vi "parse core.vi"(11 "URL":string) -> (0 "query":string, 1 "path":string, 2 "port":string, 3 "host":string, 4 "password":string, 5 "username":string, 6 "fragment":string, 7 "scheme":string)   [LabVIEW 2013, in "uniform resource locator.lvlib"]
uses:
  uniform resource locator.lvlib
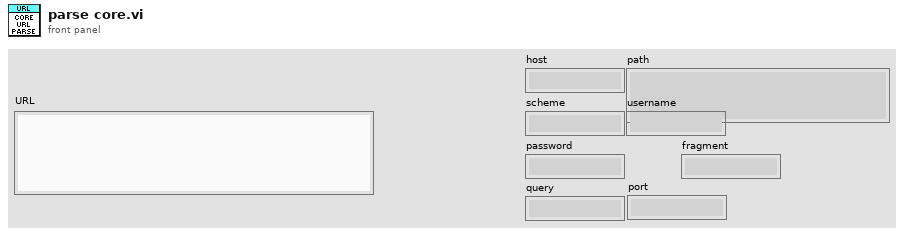
[diagram p1: front panel]
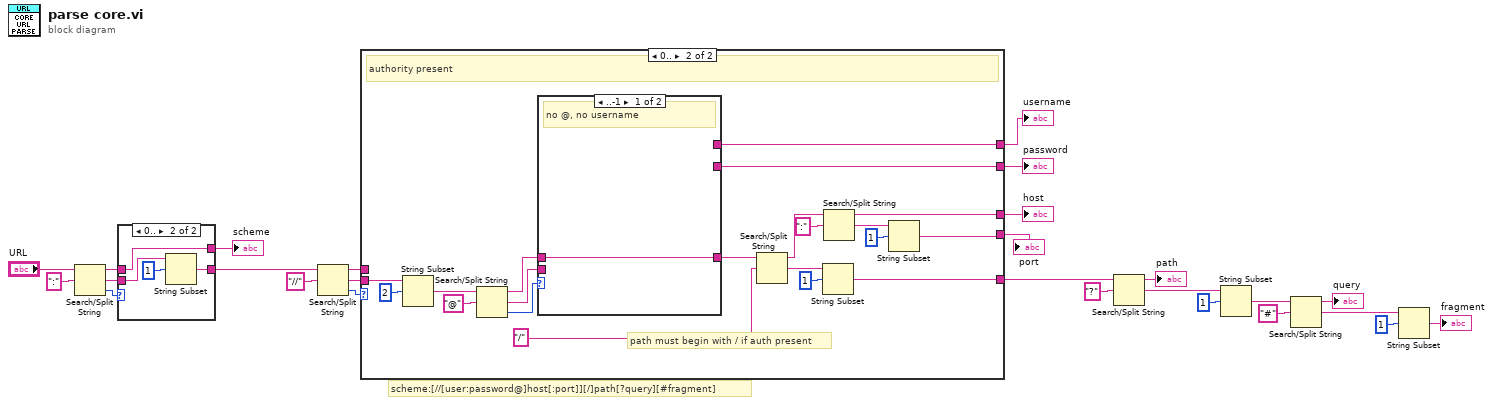
[diagram p0: block diagram]
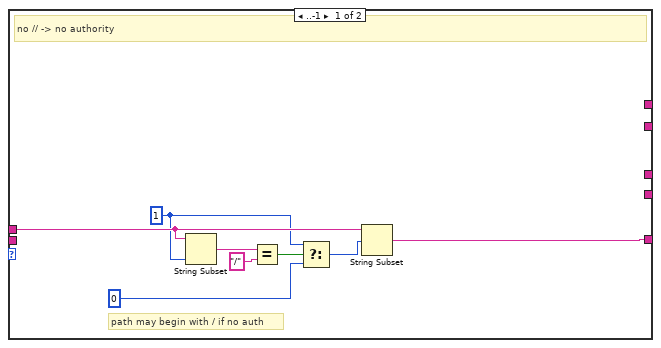
[diagram p2: hidden frame]
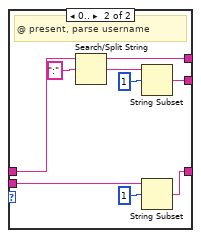
[diagram p3: hidden frame]
diagram:
  # "scheme:[//[user:password@]host[:port]][/]path[?query][#fragment]"
  n1 = Search/Split String(string="URL", search string/char (-)=":" ("regular expression")) -> (substring before match=w22:string, match + rest of string=w21:string, offset of match=w24:i32)  [unwired: 1 in]
  n2 = case shown="0.." w24 {
    tunnel: [_ w31] -> w23
    tunnel: w22 -> [w27 w31]
    tunnel: [w27 w29] -> w17
    tunnel: w21 -> [_ w30]
    frame ..-1 {
    }
    frame 0.. {
      n3 = String Subset(string=w30, offset (0)=1) -> (substring=w29:string)  [unwired: 1 in]
    }
  }
  "scheme" <- w23
  n4 = Search/Split String(string=w17, search string/char (-)="//" ("regular expression")) -> (substring before match=w19:string, match + rest of string=w20:string, offset of match=w16:i32)  [unwired: 1 in]
  n5 = case shown="0.." w16 {
    tunnel: w20 -> [_ w59]
    tunnel: w19 -> [w37 _]
    tunnel: [_ w44] -> w15
    tunnel: [w36 w47] -> w9
    tunnel: [_ w52] -> w14
    tunnel: [_ w51] -> w13
    tunnel: [_ w40] -> w1
    frame ..-1 {
      w34 = 1 ("length (rest)")
      # "path may begin with / if no auth"
      # "no // -> no authority"
      n6 = String Subset(string=w37, length (rest)=w34) -> (substring=w39:string)  [unwired: 1 in]
      n7 = Equal?(x=w39, y="/" ("regular expression")) -> (x = y?=w35:bool)
      n8 = Select(t=w34, s=w35, f=0) -> (s? t:f=w32:i32)
      n9 = String Subset(string=w37, offset (0)=w32) -> (substring=w36:string)  [unwired: 1 in]
    }
    frame 0.. {
      # "path must begin with / if auth present"
      # "authority present"
      n10 = String Subset(string=w59, offset (0)=2) -> (substring=w54:string)  [unwired: 1 in]
      n11 = Search/Split String(string=w54, search string/char (-)="@" ("regular expression")) -> (substring before match=w56:string, match + rest of string=w55:string, offset of match=w57:i32)  [unwired: 1 in]
      n12 = case shown="..-1" w57 {
        tunnel: w56 -> [w60 w64]
        tunnel: [w60 w68] -> w48
        tunnel: w55 -> [_ w69]
        tunnel: [_ w62] -> w52
        tunnel: [_ w61] -> w51
        frame ..-1 {
          # "no @, no username"
        }
        frame 0.. {
          # "@ present, parse username"
          n13 = Search/Split String(string=w64, search string/char (-)=":" ("regular expression")) -> (substring before match=w62:string, match + rest of string=w66:string)  [unwired: 1 in, 1 out]
          n14 = String Subset(string=w66, offset (0)=1) -> (substring=w61:string)  [unwired: 1 in]
          n15 = String Subset(string=w69, offset (0)=1) -> (substring=w68:string)  [unwired: 1 in]
        }
      }
      n16 = Search/Split String(string=w48, search string/char (-)="/" ("regular expression")) -> (substring before match=w42:string, match + rest of string=w50:string)  [unwired: 1 in, 1 out]
      n17 = String Subset(string=w50, offset (0)=1) -> (substring=w47:string)  [unwired: 1 in]
      n18 = Search/Split String(string=w42, search string/char (-)=":" ("regular expression")) -> (substring before match=w44:string, match + rest of string=w45:string)  [unwired: 1 in, 1 out]
      n19 = String Subset(string=w45, offset (0)=1) -> (substring=w40:string)  [unwired: 1 in]
    }
  }
  "host" <- w15
  "username" <- w14
  "password" <- w13
  "port" <- w1
  n20 = Search/Split String(string=w9, search string/char (-)="?" ("regular expression")) -> (substring before match=→"path":string, match + rest of string=w10:string)  [unwired: 1 in, 1 out]
  n21 = String Subset(string=w10, offset (0)=1) -> (substring=w4:string)  [unwired: 1 in]
  n22 = Search/Split String(string=w4, search string/char (-)="#" ("regular expression")) -> (substring before match=→"query":string, match + rest of string=w6:string)  [unwired: 1 in, 1 out]
  n23 = String Subset(string=w6, offset (0)=1) -> (substring=→"fragment":string)  [unwired: 1 in]
